vi "CAN BL Init.vi"(7 "pCmdList":T1, 8 "error in (no error)":errorcluster, 9 "pInitConfig":T2, 10 "CANIndex":i32, 11 "DevHandle":i32) -> (0 "error out":errorcluster, 1 "pInitConfig out":T2, 3 "function return":i32, 5 "pCmdList out":T1)   [LabVIEW 2010, in "usb2an.lvlib"]
doc: "int WINAPI CAN_BL_Init(int DevHandle,int CANIndex,PCAN_INIT_CONFIG pInitConfig,PCBL_CMD_LIST pCmdList);"
uses:
  usb2an.lvlib
  USB2XXX.dll
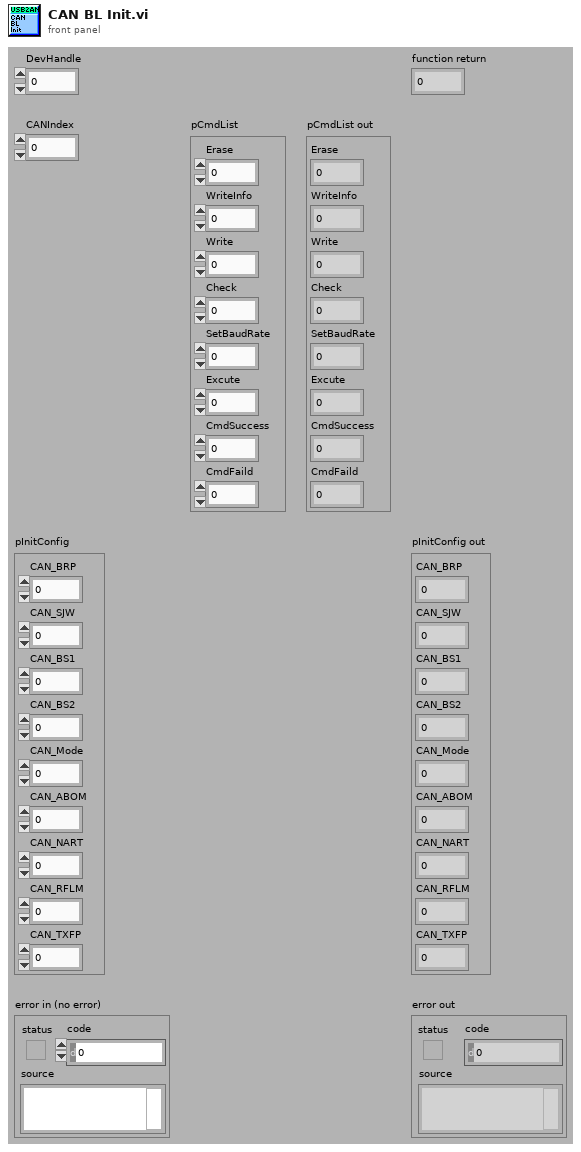
[diagram p1: front panel]
types:
  T1 = cluster{"Erase":u8, "WriteInfo":u8, "Write":u8, "Check":u8, "SetBaudRate":u8, "Excute":u8, "CmdSuccess":u8, "CmdFaild":u8}
  T2 = cluster{"CAN_BRP":u32, "CAN_SJW":u8, "CAN_BS1":u8, "CAN_BS2":u8, "CAN_Mode":u8, "CAN_ABOM":u8, "CAN_NART":u8, "CAN_RFLM":u8, "CAN_TXFP":u8}
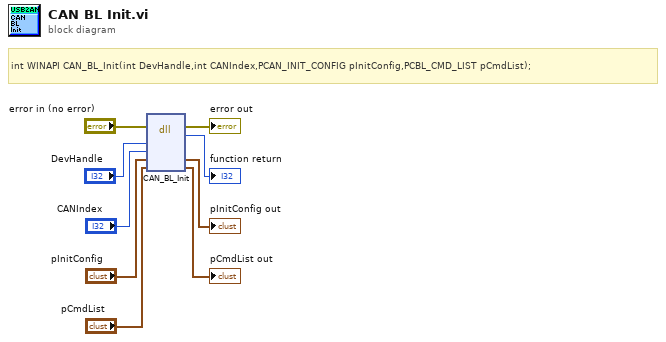
[diagram p0: block diagram]
diagram:
  # "int WINAPI CAN_BL_Init(int DevHandle,int CANIndex,PCAN_INIT_CONFIG pInitConfig,PCBL_CMD_LIST pCmdList);"
  n1 = dll-call lib="E:/OtherWork/STM32/USB2XXX_Example/sdk/api/Labview/USB2XXX.*" fn="CAN_BL_Init"(error in="error in (no error)", "DevHandle"="DevHandle", "CANIndex"="CANIndex", "pInitConfig"="pInitConfig", "pCmdList"="pCmdList") -> (error out=→"error out":errorcluster, →"function return":i32, "pInitConfig"=→"pInitConfig out":T2, "pCmdList"=→"pCmdList out":T1)  [unwired: 4 in, 1 out]
